vi "Header Footer column.vi"(7 "Header or Footer":T2, 8 "error in (no error)":errorcluster, 9 "numColumns":i32, 10 "Page points":T3={"Start at page"=612, "Orientation"=enum."Landscape", "widht"=70.86614, "height"=70.86614, "Margin left"=70.86614, "Margin right"=70.86614, "Margin top"=72.0, "Margin bottom"=72.0}) -> (0 "error out":errorcluster, 1 "Table Column":dbl[](array[numeric]), 2 "Table position":T1)   [LabVIEW 2012]
doc: "Version 1.0\nDeveloped by Jean-Marc Simard\nCopyright © 2010, Exaprom Inc.\nAll rights reserved.\nLicense: BSD\n\nWith iTextSharp 4.1.6 (http://itextsharp.sourceforge.net)\nunder Mozilla Public License Version 1.1\n(http://www.mozilla.org/MPL/MPL-1.1.html)"
uses:
  Controls/Page dimensions.ctl
  Controls/Page Orientation.ctl
  Controls/Header or Footer.ctl
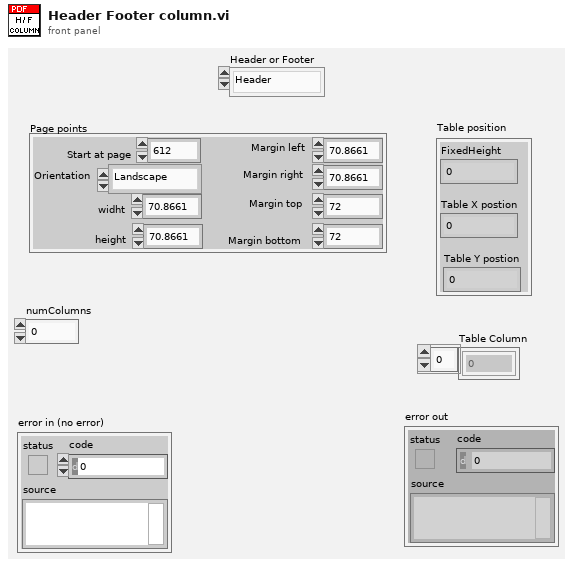
[diagram p1: front panel]
types:
  T1 = cluster{"FixedHeight":dbl, "Table X postion":dbl, "Table Y postion":dbl}
  T2 = typedef "Header or Footer.ctl" = enum16{"Header", "Footer"}
  T3 = typedef "Page dimensions.ctl" = cluster{"Start at page":i32, "Orientation":T4, "widht":sgl, "height":sgl, "Margin left":sgl, "Margin right":sgl, "Margin top":sgl, "Margin bottom":sgl}
  T4 = typedef "Page Orientation.ctl" = enum16{"Portrait", "Landscape"}
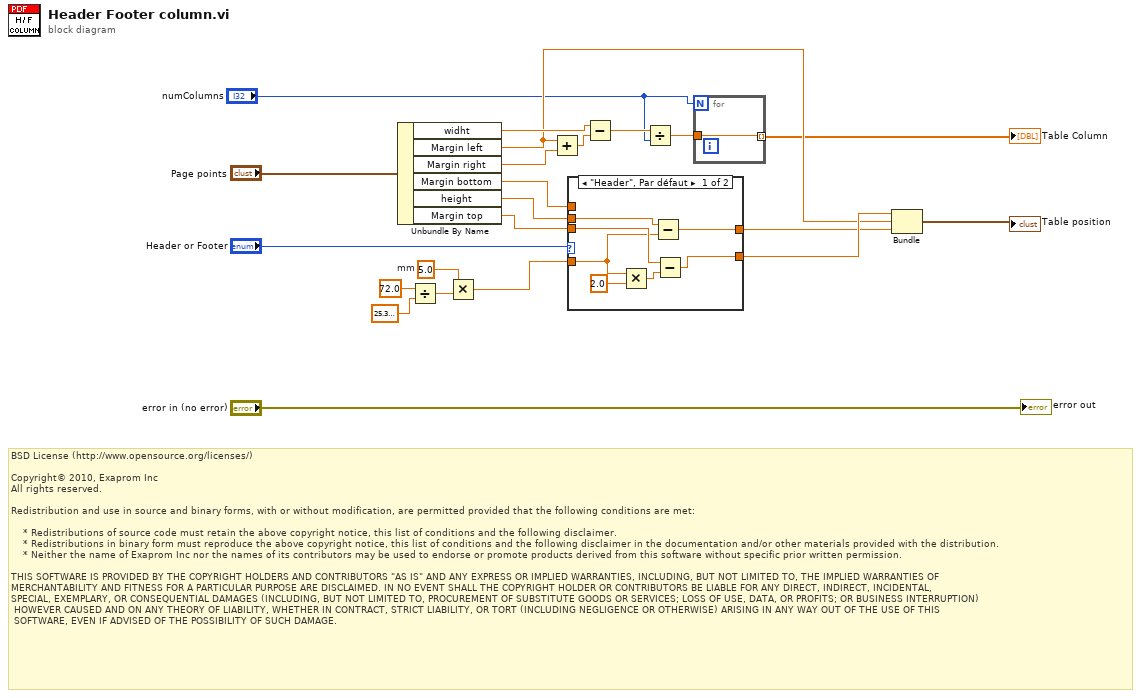
[diagram p0: block diagram]
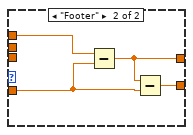
[diagram p2: hidden frame]
diagram:
  w13 = sgl 5.0  # mm
  # "BSD License (http://www.opensource.org/licenses/)\n\nCopyright© 2010, Exaprom Inc\nAll rights reserved.\n\nRedistribution and use in source and binary forms, with or without modification, are permitted provided that the following conditions are met:\n\n    * Redistributions of source code must retain the above copyright notice, this list of conditions and the following disclaimer.\n    * Redistributions in binary form must reproduce the above copyright notice, this list of conditions and the following disclaimer in the documentation and/or other materials provided with the distribution.\n    * Neither the name of Exaprom Inc nor the names of its contributors may be used to endorse or promote products derived from this software without specific prior written permission.\n\nTHIS SOFTWARE IS PROVIDED BY THE COPYRIGHT HOLDERS AND CONTRIBUTORS \"AS IS\" AND ANY EXPRESS OR IMPLIED WARRANTIES, INCLUDING, BUT NOT LIMITED TO, THE IMPLIED WARRANTIES OF \nMERCHANTABILITY AND FITNESS FOR A PARTICULAR PURPOSE ARE DISCLAIMED. IN NO EVENT SHALL THE COPYRIGHT HOLDER OR CONTRIBUTORS BE LIABLE FOR ANY DIRECT, INDIRECT, INCIDENTAL,\nSPECIAL, EXEMPLARY, OR CONSEQUENTIAL DAMAGES (INCLUDING, BUT NOT LIMITED TO, PROCUREMENT OF SUBSTITUTE GOODS OR SERVICES; LOSS OF USE, DATA, OR PROFITS; OR BUSINESS INTERRUPTION)\n HOWEVER CAUSED AND ON ANY THEORY OF LIABILITY, WHETHER IN CONTRACT, STRICT LIABILITY, OR TORT (INCLUDING NEGLIGENCE OR OTHERWISE) ARISING IN ANY WAY OUT OF THE USE OF THIS\n SOFTWARE, EVEN IF ADVISED OF THE POSSIBILITY OF SUCH DAMAGE."
  n1 = Unbundle By Name("Page points") -> ("widht"=w20:sgl, "Margin left"=w7:sgl, "Margin right"=w19:sgl, "Margin bottom"=w17:sgl, "height"=w10:sgl, "Margin top"=w9:sgl)
  n2 = Divide(x=sgl 72.0, y=sgl 25.4) -> (x/y=w14:sgl)
  n3 = Multiply(x=w13, y=w14) -> (x*y=w12:sgl)
  n4 = Add(x=w7, y=w19) -> (x+y=w22:sgl)
  n5 = case shown="\"Header\", Par défaut" "Header or Footer" {
    tunnel: w17 -> [_ w33]
    tunnel: w12 -> [w25 w31]
    tunnel: [w28 w32] -> w6
    tunnel: w10 -> [w29 _]
    tunnel: w9 -> [w27 _]
    tunnel: [w23 w30] -> w8
    frame "Header", Default {
      n6 = Multiply(x=w25, y=sgl 2.0) -> (x*y=w26:sgl)
      n7 = Subtract(x=w29, y=w25) -> (x-y=w28:sgl)
      n8 = Subtract(x=w27, y=w26) -> (x-y=w23:sgl)
    }
    frame "Footer" {
      n9 = Subtract(x=w33, y=w31) -> (x-y=w32:sgl)
      n10 = Subtract(x=w32, y=w31) -> (x-y=w30:sgl)
    }
  }
  n11 = Subtract(x=w20, y=w22) -> (x-y=w21:sgl)
  n12 = Divide(x=w21, y="numColumns") -> (x/y=w2:sgl)
  n13 = for {
    N: "numColumns" -> [_]
    tunnel: w2 -> [w34]
    tunnel: [w34] -> w1 mode=indexing
  }
  "Table Column" <- w1
  n14 = Bundle(w8, "Margin left"=w7, w6) -> (→"Table position":cluster{sgl, "Margin left":sgl, sgl})  [unwired: 1 out]
  "error out" <- "error in (no error)"
